vi "Read Dataset.vi"(8 "error in (no error)":errorcluster, 11 "Saving Path":path) -> (0 "error out":errorcluster, 3 "Information":T1)   [LabVIEW 2020]
uses:
  <vilib>/Utility/config.llb/Read Key (Double).vi
  <vilib>/Utility/config.llb/Read Key (Boolean).vi
  <vilib>/Utility/config.llb/Read Key (String).vi
  <vilib>/Utility/config.llb/Read Key (Path).vi
  <vilib>/Utility/config.llb/NI_LVConfig.lvlib
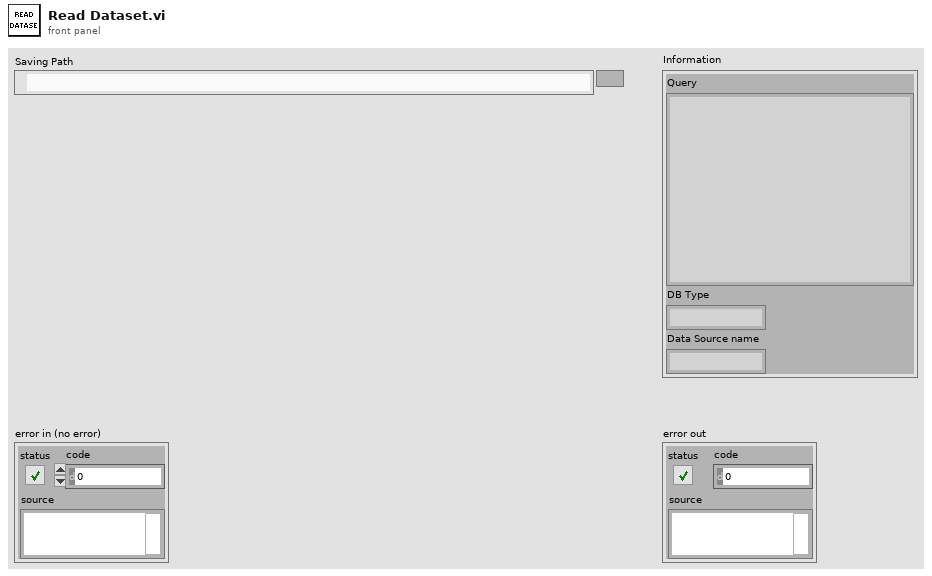
[diagram p1: front panel]
types:
  T1 = cluster{"Query":string, "DB Type":string, "Data Source name":string}
  T2 = typedef "NI_LVConfig.lvlib/Config Data RefNum.ctl" = refnum<k1>
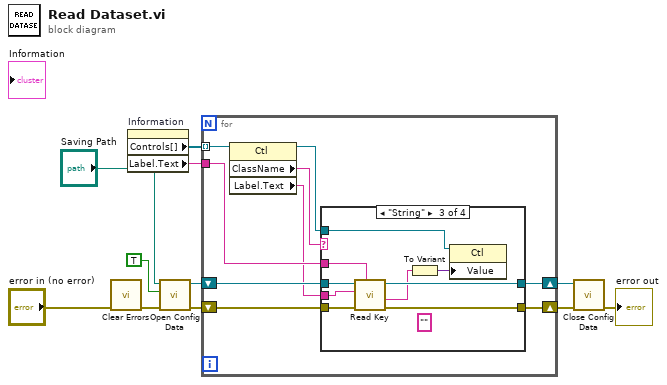
[diagram p0: block diagram]
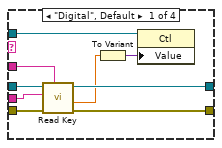
[diagram p2: hidden frame]
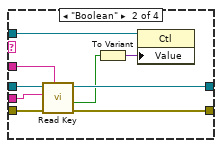
[diagram p3: hidden frame]
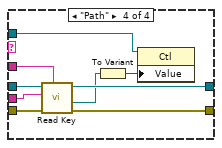
[diagram p4: hidden frame]
diagram:
  n1 = call <vilib>:"Clear Errors.vi"("error in (no error)"="error in (no error)") -> ("error out"=w1:errorcluster)  [unwired: 5 in, 1 out]
  n2 = property on="Information" class="Clust (strict)"() -> ("Controls[]"=w3:refnum<vi>[], "Label.Text"=w4:string)  [unwired: 2 in, 2 out]
  n3 = call <vilib>:"Open Config Data.vi"("error in (no error)"=w1, "create file if necessary (T)"=TRUE, "configuration file path"="Saving Path") -> ("error out"=w7:errorcluster, "refnum"=w6:T2)  [unwired: 6 in, 1 out]
  n4 = for {
    shift-right: [w15] -> w9
    shift-left: w7 -> [w17]
    shift-right: [w14] -> w8
    shift-left: w6 -> [w16]
    tunnel: w4 -> [w18]
    tunnel: w3 -> [w20] mode=indexing
    n5 = property class="Ctl"(reference=w20) -> (reference out=w12:refnum<vi>, "ClassName"=w19:string, "Label.Text"=w13:string)  [unwired: 1 in, 1 out]
    n6 = case shown="\"String\"" w19 {
      tunnel: w18 -> [w26 w32 w47 w56]
      tunnel: w17 -> [w29 w35 w43 w52]
      tunnel: w16 -> [w25 w38 w46 w55]
      tunnel: [w28 w37 w45 w54] -> w15
      tunnel: [w27 w36 w44 w53] -> w14
      tunnel: w13 -> [w24 w34 w42 w51]
      tunnel: w12 -> [w21 w30 w39 w50]
      frame "Digital", Default {
        n7 = call-poly <vilib>:"Read Key.vi"("section"=w26, "error in (no error)"=w29, "key"=w24, "refnum"=w25) -> ("error out"=w28:errorcluster, "value"=w22:dbl, "refnum out"=w27:T2)  [unwired: 4 in, 1 out]
        n8 = To Variant(anything=w22) -> (Variant=w23:variant)
        n9 = property class="Ctl"(reference=w21, "Value"=w23) -> ()  [unwired: 1 in, 2 out]
      }
      frame "Boolean" {
        n10 = call-poly <vilib>:"Read Key.vi"("section"=w32, "error in (no error)"=w35, "key"=w34, "refnum"=w38) -> ("error out"=w37:errorcluster, "value"=w31:bool, "refnum out"=w36:T2)  [unwired: 4 in, 1 out]
        n11 = To Variant(anything=w31) -> (Variant=w33:variant)
        n12 = property class="Ctl"(reference=w30, "Value"=w33) -> ()  [unwired: 1 in, 2 out]
      }
      frame "String" {
        (unwired) ""
        n13 = call-poly <vilib>:"Read Key.vi"("section"=w47, "error in (no error)"=w43, "key"=w42, "refnum"=w46) -> ("error out"=w45:errorcluster, "value"=w40:string, "refnum out"=w44:T2)  [unwired: 4 in, 1 out]
        n14 = To Variant(anything=w40) -> (Variant=w41:variant)
        n15 = property class="Ctl"(reference=w39, "Value"=w41) -> ()  [unwired: 1 in, 2 out]
      }
      frame "Path" {
        n16 = call-poly <vilib>:"Read Key.vi"("section"=w56, "error in (no error)"=w52, "key"=w51, "refnum"=w55) -> ("error out"=w54:errorcluster, "value"=w49:path, "refnum out"=w53:T2)  [unwired: 4 in, 1 out]
        n17 = To Variant(anything=w49) -> (Variant=w48:variant)
        n18 = property class="Ctl"(reference=w50, "Value"=w48) -> ()  [unwired: 1 in, 2 out]
      }
    }
  }
  n19 = call <vilib>:"Close Config Data.vi"("error in (no error)"=w9, "refnum"=w8) -> ("error out"=→"error out":errorcluster)  [unwired: 8 in, 1 out]
